vi "ACP_Display_Helper.vi"(6 "Min":sgl, 7 "Mask":dbl[](array[numeric]), 8 "RR":dbl, 9 "RL":dbl, 10 "LR":dbl, 11 "LL":dbl) -> (5 "Mask_Out":dbl[](array[numeric]))   [LabVIEW 2014]
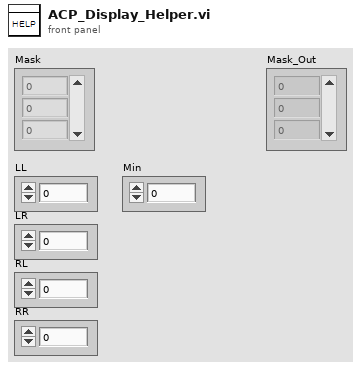
[diagram p1: front panel]
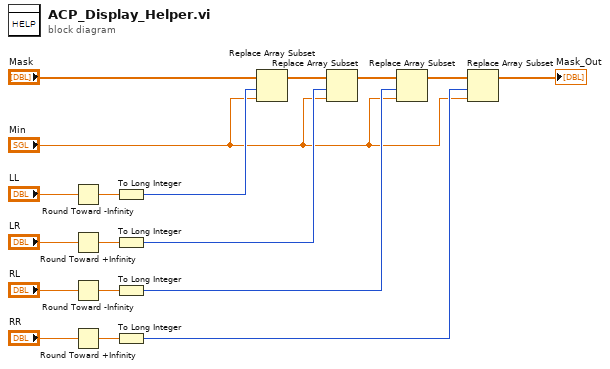
[diagram p0: block diagram]
diagram:
  n1 = Round Toward -Infinity(1:"LL") -> (0:w14:dbl)
  n2 = Round Toward +Infinity(x="LR") -> (ceil(x): smallest int >= x=w11:dbl)
  n3 = Round Toward -Infinity(1:"RL") -> (0:w12:dbl)
  n4 = Round Toward +Infinity(x="RR") -> (ceil(x): smallest int >= x=w13:dbl)
  n5 = To Long Integer(number=w14) -> (32bit integer=w9:i32)
  n6 = To Long Integer(number=w11) -> (32bit integer=w4:i32)
  n7 = To Long Integer(number=w12) -> (32bit integer=w3:i32)
  n8 = To Long Integer(number=w13) -> (32bit integer=w2:i32)
  n9 = Replace Array Subset(array="Mask", new element="Min", index=w9) -> (w8:dbl[])
  n10 = Replace Array Subset(array=w8, new element="Min", index=w4) -> (w7:dbl[])
  n11 = Replace Array Subset(array=w7, new element="Min", index=w3) -> (w6:dbl[])
  n12 = Replace Array Subset(array=w6, new element="Min", index=w2) -> (→"Mask_Out":dbl[])
